vi "_Set Target Object (Comm).vi"(8 "error in (no error)":errorcluster, 10 "Target Object":refnum<class "Interfaceable.lvclass">, 11 "Interface in":refnum<class "IUnknown.lvclass">) -> (0 "error out":errorcluster, 3 "Interface out":refnum<class "IUnknown.lvclass">)   [LabVIEW 2009, in "IUnknown.lvclass"]
doc: "Provides an implementation for injecting a target object into an Interface. This vi is used only by Interfaceable:_GetInterface."
uses:
  IUnknown.lvclass
  Interfaceable Class/Interfaceable.lvclass
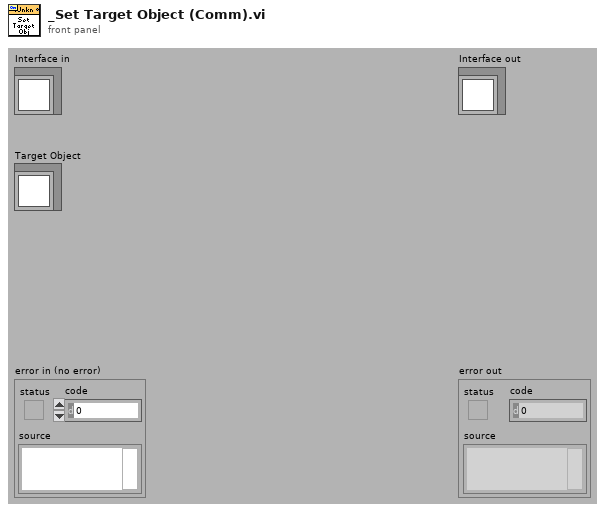
[diagram p1: front panel]
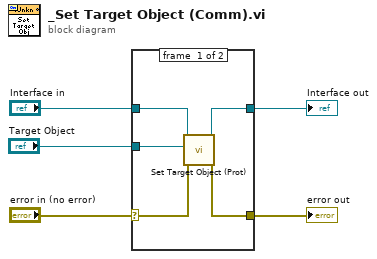
[diagram p0: block diagram]
diagram:
  n1 = case shown="No Error" "error in (no error)" {
    selector: "error in (no error)" -> [w8 w12]
    tunnel: [w7 w12] -> w4
    tunnel: [w9 w11] -> w2
    tunnel: "Interface in" -> [w10 w11]
    tunnel: "Target Object" -> [w6 _]
    frame #0 {
      n2 = call "Set Target Object (Prot).vi"("error in (no error)"=w8, "Target Object"=w6, "IUnknown in"=w10) -> ("error out"=w7:errorcluster, "IUnknown out"=w9:refnum<class "IUnknown.lvclass">)  [unwired: 7 in]
    }
    frame #1 {
    }
  }
  "error out" <- w4
  "Interface out" <- w2
